vi "Boolean to String.vi"(0 "BooleanValue":bool) -> (1 "StringForm":string, 2 "BackgroundColor":u32)   [LabVIEW 2016, in "M1M3SupportEUI_Views.lvlib"]
uses:
  M1M3SupportEUI_Views.lvlib
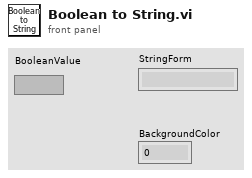
[diagram p1: front panel]
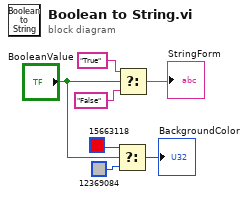
[diagram p0: block diagram]
diagram:
  n1 = Select(t=u32 15663118, s="BooleanValue", f=u32 12369084) -> (s? t:f=→"BackgroundColor":u32)
  n2 = Select(t="True", s="BooleanValue", f="False") -> (s? t:f=→"StringForm":string)
